vi "Convolution.vi"(8 "Bias":dbl[](array[numeric]), 9 "Convolution Settings":T1={"Stride"=3, "Offset - x"=0, "Offset - y"=0, "Size Mode"=enum."Round Up"}, 10 "Kernals":cluster{"Kernal":dbl[][][]}[](array[cluster]), 11 "Data In":dbl[][][](array[numeric])) -> (3 "Data Out":dbl[][][](array[numeric]))   [LabVIEW 2015]
panel:
  out "Array":dbl[][][](array[numeric])
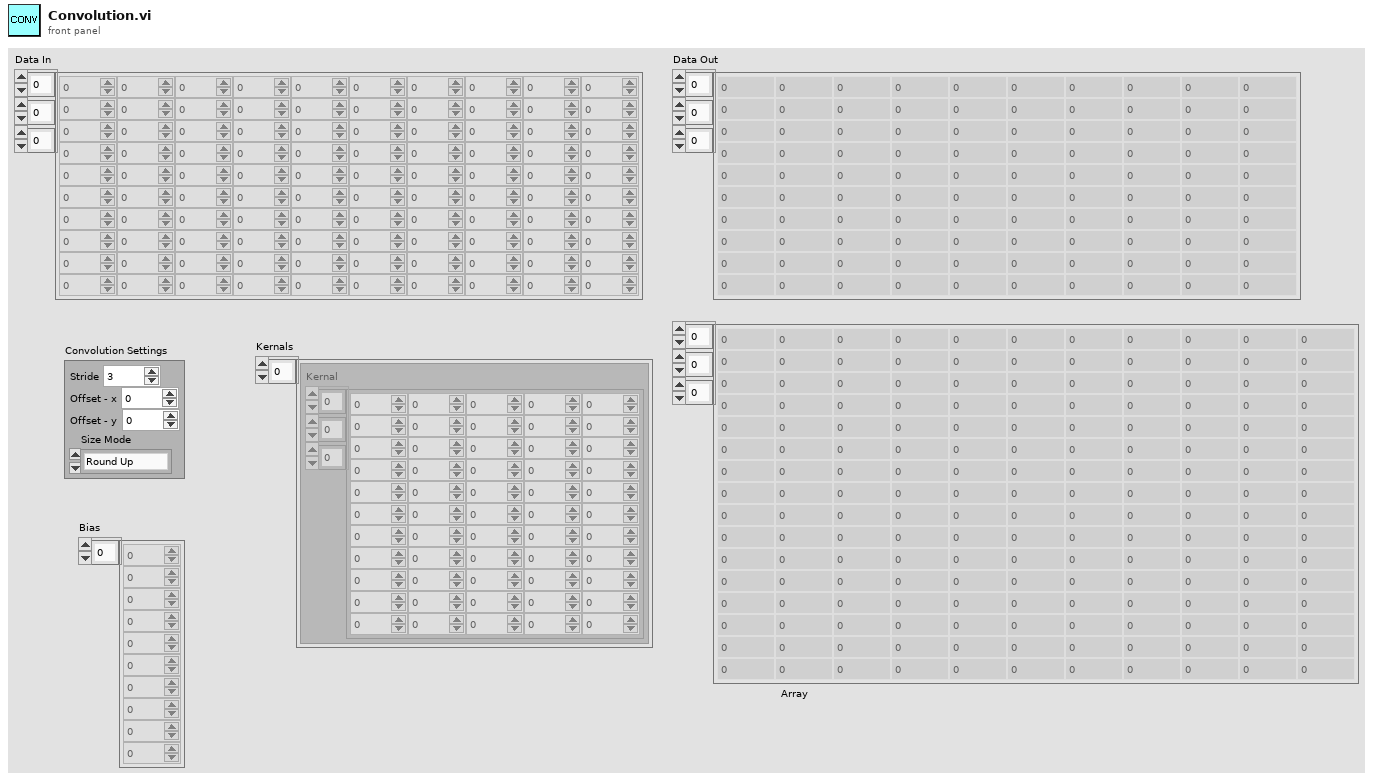
[diagram p1: front panel]
types:
  T1 = cluster{"Stride":i32, "Offset - x":i32, "Offset - y":i32, "Size Mode":enum16{"Round Up", "Round Down", "Same"}}
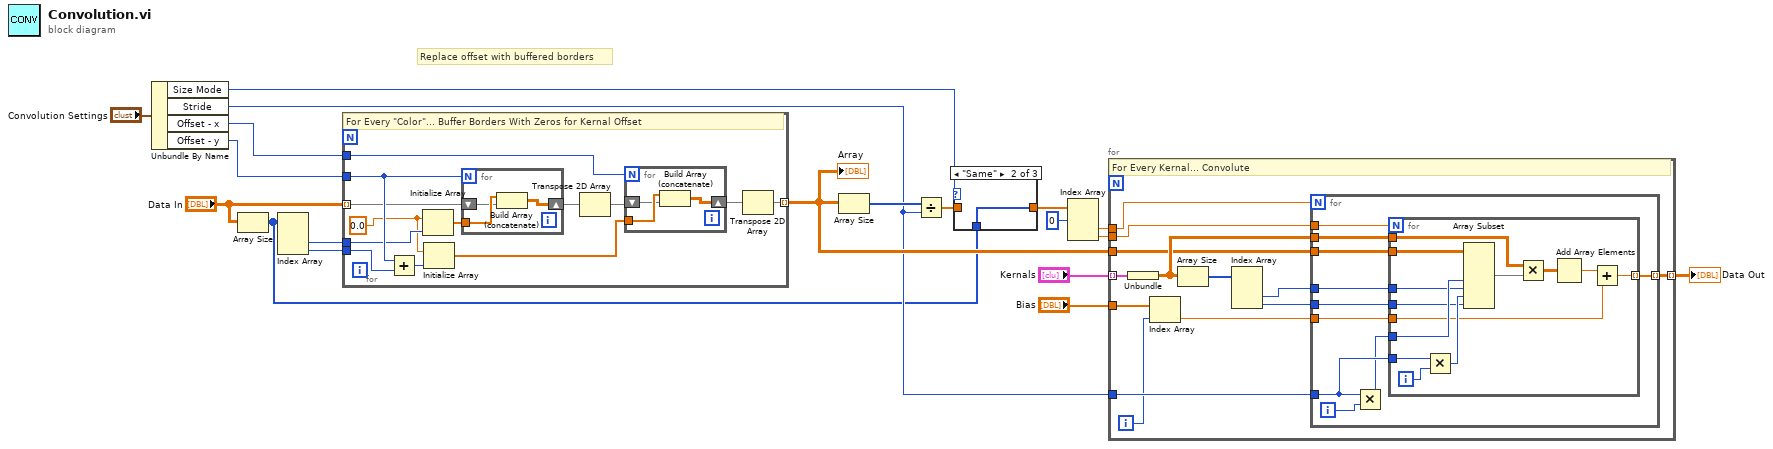
[diagram p0: block diagram]
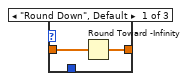
[diagram p2: hidden frame]
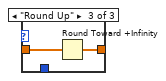
[diagram p3: hidden frame]
diagram:
  # "Replace offset with buffered borders"
  n1 = Unbundle By Name("Convolution Settings") -> ("Size Mode"=w6:enum16{"Round Up", "Round Down", "Same"}, "Stride"=w7:i32, "Offset - x"=w9:i32, "Offset - y"=w8:i32)
  n2 = Array Size(array="Data In") -> (size(s)=w1:i32[])
  n3 = Index Array(array=w1) -> (element #2=w3:i32, element #3=w2:i32)  [unwired: 3 in, 1 out]
  n4 = for {
    tunnel: w8 -> [w24]
    tunnel: "Data In" -> [w21] mode=indexing
    tunnel: [w29] -> w13 mode=indexing
    tunnel: w9 -> [w26]
    tunnel: w3 -> [w22]
    tunnel: w2 -> [w23]
    w20 = 0.0 ("element")
    # "For Every \"Color\"... Buffer Borders With Zeros for Kernal Offset"
    n5 = Add(x=w24, y=w23) -> (x+y=w32:i32)
    n6 = Initialize Array(w20, w22) -> (w31:dbl[])
    n7 = Initialize Array(w20, w32) -> (w27:dbl[])
    n8 = for {
      N: w24 -> [_]
      tunnel: w31 -> [w38]
      shift-right: [w36] -> w30
      shift-left: w21 -> [w37]
      n9 = Build Array (concatenate)(w38, w37) -> (w36:dbl[][])
    }
    n10 = Transpose 2D Array(2D array=w30) -> (transposed array=w28:dbl[][])
    n11 = for {
      N: w26 -> [_]
      tunnel: w27 -> [w35]
      shift-right: [w33] -> w25
      shift-left: w28 -> [w34]
      n12 = Build Array (concatenate)(w35, w34) -> (w33:dbl[][])
    }
    n13 = Transpose 2D Array(2D array=w25) -> (transposed array=w29:dbl[][])
  }
  "Array" <- w13
  n14 = Array Size(array=w13) -> (size(s)=w14:i32[])
  n15 = Divide(x=w14, y=w7) -> (x/y=w15:dbl[])
  n16 = case shown="\"Same\"" w6 {
    tunnel: [w39 w41 w43] -> w16
    tunnel: w15 -> [w40 _ w42]
    tunnel: w1 -> [_ w41 _]
    frame "Round Down", Default {
      n17 = Round Toward -Infinity(1:w40) -> (0:w39:dbl[])
    }
    frame "Same" {
    }
    frame "Round Up" {
      n18 = Round Toward +Infinity(x=w42) -> (ceil(x): smallest int >= x=w43:dbl[])
    }
  }
  n19 = Index Array(array=w16, index #1=0 ("index")) -> (element #2=w12:dbl, element #3=w11:dbl)  [unwired: 2 in, 1 out]
  n20 = for {
    tunnel: w13 -> [w54]
    tunnel: w7 -> [w52]
    tunnel: "Kernals" -> [w56] mode=indexing
    tunnel: [w53] -> w18 mode=indexing
    tunnel: w12 -> [w51]
    tunnel: w11 -> [w50]
    tunnel: "Bias" -> [w46]
    i -> [w45]
    # "For Every Kernal... Convolute"
    n21 = Unbundle(w56) -> ("Kernal"=w55:dbl[][][])
    n22 = Index Array(array=w46, index=w45) -> (element=w44:dbl)
    n23 = Array Size(array=w55) -> (size(s)=w49:i32[])
    n24 = Index Array(array=w49) -> (element #2=w48:i32, element #3=w47:i32)  [unwired: 3 in, 1 out]
    n25 = for {
      N: w51 -> [_]
      tunnel: w50 -> [w66]
      tunnel: w52 -> [w64]
      tunnel: w55 -> [w62]
      tunnel: w54 -> [w61]
      tunnel: [w60] -> w53 mode=indexing
      tunnel: w48 -> [w59]
      tunnel: w47 -> [w58]
      tunnel: w44 -> [w57]
      i -> [w65]
      n26 = Multiply(x=w64, y=w65) -> (x*y=w63:i32)
      n27 = for {
        N: w66 -> [_]
        tunnel: w64 -> [w78]
        tunnel: w63 -> [w77]
        tunnel: w62 -> [w74]
        tunnel: w61 -> [w76]
        tunnel: [w67] -> w60 mode=indexing
        tunnel: w59 -> [w71]
        tunnel: w58 -> [w70]
        tunnel: w57 -> [w69]
        i -> [w79]
        n28 = Multiply(x=w78, y=w79) -> (x*y=w72:i32)
        n29 = Array Subset(array=w76, index (dim 1)=w77, length (dim 1)=w71, index (dim 2)=w72, length (dim 2)=w70) -> (w75:dbl[][][])  [unwired: 2 in]
        n30 = Multiply(x=w74, y=w75) -> (x*y=w73:dbl[][][])
        n31 = Add Array Elements(numeric array=w73) -> (sum=w68:dbl)
        n32 = Add(x=w68, y=w69) -> (x+y=w67:dbl)
      }
    }
  }
  "Data Out" <- w18
